vi "Terminal-PressureSystem-LoadingUnit-ParametersSetter.vi"(8 "error in (no error)":errorcluster caption="错误输入（无错误）", 9 "轴向液压缸加载力":u16, 10 "径向液压缸加载力":u16, 11 "write operation timeout (ms)":i32=5000 caption="写操作超时（5000毫秒）") -> (0 "error out":errorcluster caption="错误输出")   [LabVIEW 2014]
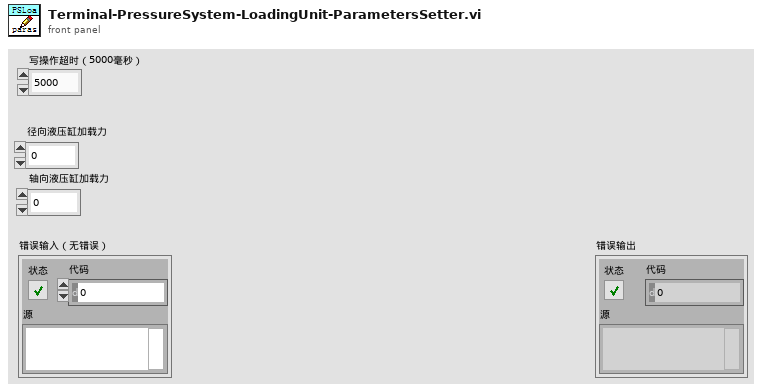
[diagram p1: front panel]
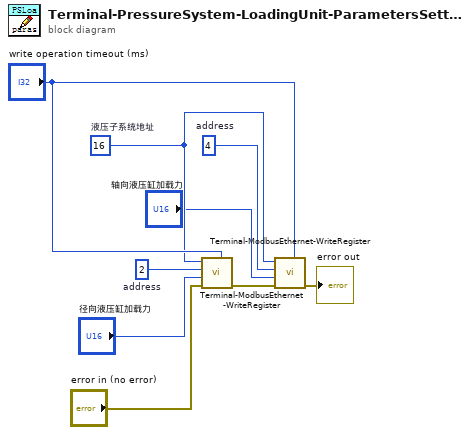
[diagram p0: block diagram]
diagram:
  w2 = u16 4  # address
  w4 = u16 2  # address
  w5 = u8 16  # 液压子系统地址
  n1 = call "Terminal-ModbusEthernet-WriteRegister.vi"("write operation timeout (ms)"="write operation timeout (ms)", "error in"="error in (no error)", "holding register value"="径向液压缸加载力", "address"=w4, "unit ID"=w5) -> ("error out"=w7:errorcluster)  [unwired: 6 in]
  n2 = call "Terminal-ModbusEthernet-WriteRegister.vi"("write operation timeout (ms)"="write operation timeout (ms)", "error in"=w7, "holding register value"="轴向液压缸加载力", "address"=w2, "unit ID"=w5) -> ("error out"=→"error out":errorcluster)  [unwired: 6 in]
